vi "fpga_ARC Core.vi"(0 "data input":i32, 1 "ARC Constants":T2={"bufsize"=512, "bufsize-1"=511, "NChan"=8, "NChan-1"=7, "1/2SymPeriods"=10, "Neg1/2SymPeriods"=-10, "polyOrder-1"=4, "maxDec-1"=24}, 5 "data valid":bool, 7 "resample position [U64.16]":fxp<+,64,16>, 9 "stepsize [U64.8]":fxp<+,64,8>, 11 "position valid":bool, 12 "Ready for output":bool, 13 "Frequency":fxp<+,32,8> format="%.27g") -> (3 "FIFO timeout?":bool, 4 "resample data":T1 {"frequency" format="%.59g"; "Resample position" format="%.53g"; "even-angle signal" format="%.30g"}, 8 "muti_ch position valid?":bool, 14 "ready for input":bool, 15 "output valid":bool)   [LabVIEW 2011, in "NI_EP_Resample_FPGA.lvlib"]
uses:
  <vilib>/addons/Electrical Power/PQ/Resampling/NI_EP_Resample_FPGA.lvlib
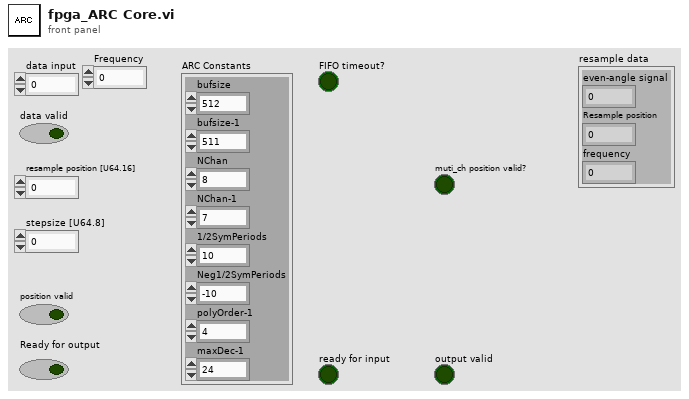
[diagram p1: front panel]
types:
  T1 = cluster{"even-angle signal":fxp<+/-,32,3>, "Resample position":fxp<+,64,16>, "frequency":fxp<+,32,8>}
  T2 = cluster{"bufsize":u16, "bufsize-1":u16, "NChan":u8, "NChan-1":u8, "1/2SymPeriods":i8, "Neg1/2SymPeriods":i8, "polyOrder-1":u8, "maxDec-1":u8}
  T3 = cluster{"sample position":u16, "coef [I32.2]":fxp<+/-,32,2>, "last tap":bool}
  T4 = cluster{"even-angle signal[I32.3]":fxp<+/-,32,3>, "resample position":fxp<+,64,16>, "frequency":fxp<+,32,8>}
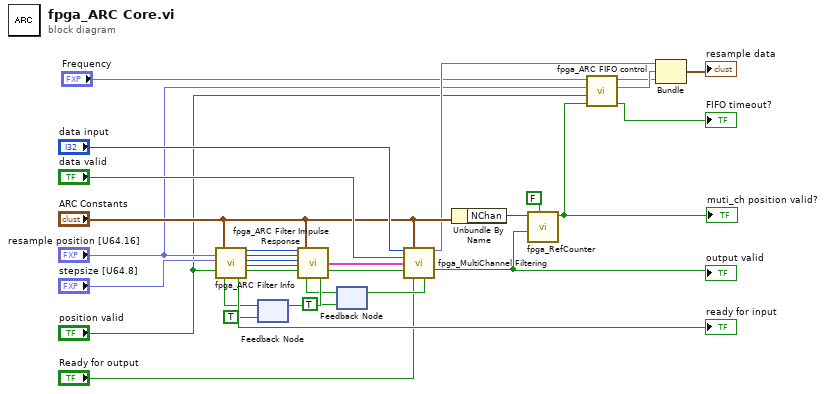
[diagram p0: block diagram]
diagram:
  n1 = feedback #1(TRUE ("ready for input")) -> (w28:bool)
  n2 = call <vilib>:"fpga_ARC Filter Info.vi"("resample position [U64.16]"="resample position [U64.16]", "stepsize [U64.8]"="stepsize [U64.8]", "input valid"="position valid", "ARC Constants"="ARC Constants", "ready for output"=w28) -> ("ready for input"=→"ready for input":bool, "Initial position"=w26:u16, "Initial offset"=w30:u32, "Number of taps"=w24:u16, "filterStepSize[U32.0]"=w29:u32, "output valid"=w25:bool)  [unwired: 1 in, 8 out]
  n3 = feedback #2(TRUE ("ready for filter")) -> (w23:bool)
  n4 = call <vilib>:"fpga_ARC Filter Impulse Response.vi"("Initial position"=w26, "Initial offset"=w30, "Number of taps"=w24, "filterStepSize[U32.0]"=w29, "input valid"=w25, "ARC Constants"="ARC Constants", "ready for output"=w23) -> ("ready for input"=w27:bool, "filter info"=w20:T3, "output valid"=w21:bool)  [unwired: 10 out]
  n5 = feedback-in #1(w27) -> ()
  n6 = call <vilib>:"fpga_MultiChannel Filtering.vi"("data input"="data input", "ARC Constants"="ARC Constants", "data valid"="data valid", "filter info"=w20, "filter valid"=w21, "Ready for output"="Ready for output") -> ("even-angle signal[I32.3]"=w11:fxp<+/-,32,3>, "output valid"=w8:bool, "ready for filter"=w22:bool)  [unwired: 7 in]
  "output valid" <- w8
  n7 = feedback-in #2(w22) -> ()
  n8 = Unbundle By Name("ARC Constants") -> ("NChan"=w10:u8)
  n9 = call <vilib>:"fpga_RefCounter.vi"("reset"=FALSE, "input valid?"=w8, "NChan"=w10) -> ("Multichannel enable"=w4:bool)  [unwired: 7 in, 1 out]
  "muti_ch position valid?" <- w4
  n10 = call <vilib>:"fpga_ARC FIFO control.vi"("Read FIFO"=w4, "write FIFO"="position valid", "resample position"="resample position [U64.16]", "frequency"="Frequency") -> ("FIFO time out?"=→"FIFO timeout?":bool, "resample position"=w3:fxp<+,64,16>, "frequency"=w2:fxp<+,32,8>)  [unwired: 5 in]
  n11 = Bundle("even-angle signal[I32.3]"=w11, "resample position"=w3, "frequency"=w2) -> (→"resample data":T4)  [unwired: 1 in]
